vi "Setup subWorkers.vi"(8 "error in":errorcluster, 11 "Server Client in":refnum<class "Server Client.lvclass">) -> (0 "error out":errorcluster, 3 "Server Client out":refnum<class "Server Client.lvclass">)   [LabVIEW 2020, in "Server Client.lvclass"]
doc: "<b>Note: Do not change the code in this VI!</b>\nThis VI performs a setup of all the statically-linked subWorkers that belong to the Worker that calls this VI. This VI is created automatically by the 'Create/Add Worker' tool and must be called <b>before</b> any statically linked subWorkers are called."
uses:
  Server Client.lvclass
  C:/Program Files (x86)/National Instruments/LabVIEW 2020/vi.lib/addons/_Workers/Library/Classes/Worker/Worker.lvclass
  subWorkers.ctl
  Listener/Listener.lvclass
  Server Client.lvclass/Server Client.ctl
  <vilib>/addons/_Workers/Library/Classes/Worker/Worker.lvclass
panel:
  out "subWorkers":T1
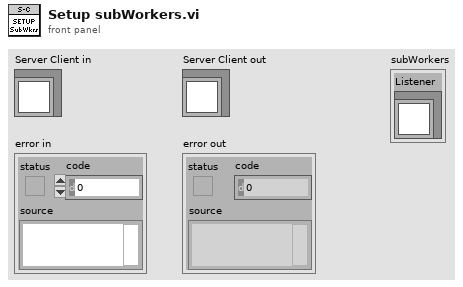
[diagram p1: front panel]
types:
  T1 = typedef "Server Client.lvclass/subWorkers.ctl" = cluster{"Listener":refnum<class "Listener.lvclass">}
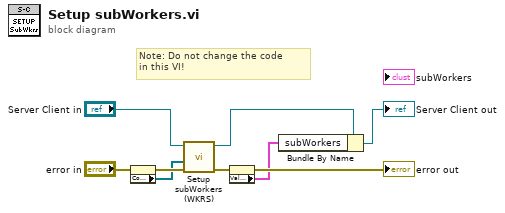
[diagram p0: block diagram]
diagram:
  # "Note: Do not change the code \nin this VI!"
  n1 = property on="subWorkers" class="Clust (strict)"(error in="error in") -> (error out=w7:errorcluster, "Controls[]"=w4:refnum<vi>[])  [unwired: 1 in, 1 out]
  n2 = call <vilib>:"Setup subWorkers (WKRS).vi"("error in"=w7, "Controls[]"=w4, "Worker"="Server Client in") -> ("error out"=w5:errorcluster, "Worker out"=w1:refnum<class "Server Client.lvclass">)  [unwired: 7 in]
  n3 = property on="subWorkers" class="Clust (strict)"(error in=w5) -> (error out=→"error out":errorcluster, "Value"=w3:T1)  [unwired: 1 in, 1 out]
  n4 = Bundle By Name(cluster=w1, "subWorkers"=w3) -> (→"Server Client out":refnum<class "Server Client.lvclass">)
